vi "lvEtherbone.test_snoop-multi.vi"() -> ()   [LabVIEW 2009, in "lvEtherbone.lvlib"]
doc: "This example performs a multiple read/write _one_ Etherbone device and does this multiple times. This can be used to determine the average time of transactions."
uses:
  lvEtherbone.lvlib
  lvEtherbone.eb_mode_t.ctl
  lvEtherbone.lveb_status_t.ctl
panel:
  out "nOfDevices":i32
  in  "ipPortsFile":path
  out "timePerIteration":dbl=6.0
  in  "nOfIterations":i32=1
  out "timed out?":bool
  out "eb_status":T1
  in  "dataW":u64[](array[numeric])=[291] format="%.0x"
  in  "modeW":T2 items=["EB_UNDEFINED"=-1, "EB_FIFO"=0, "EB_LINEAR"=1]
  in  "addressW":u64=32768 format="%.0x"
  in  "nR":i32
  in  "modeR":T2 items=["EB_UNDEFINED"=-1, "EB_FIFO"=0, "EB_LINEAR"=1]
  out "dataR":u64[](array[numeric]) format="%.0x"
  in  "addressR":u64=32768 format="%.0x"
  in  "timeout [ms]":i32=1000
  out "error out":errorcluster
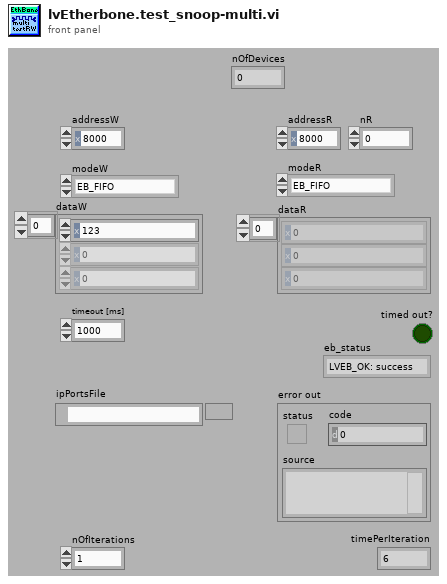
[diagram p1: front panel]
types:
  T1 = typedef "lvEtherbone.lvlib/lvEtherbone.lveb_status_t.ctl" = enum32{"LVEB_OK: success", "LVEB_UNKNOWN: unknown error", "LVEB_OS: operating system forbids access", "LVEB_PORT: port in use or unavailable", "LVEB_ID: ID invalid or out of resources", "LVEB_SOCKET: socket invalid or unavailable", "LVEB_EB: remote address is not Etherbone conformant", "LVEB_IP: bad format or network address", "LVEB_PORTWIDTH: port width error", "LVEB_DEVICEBUSY: Etherbone device still busy", "LVEB_DEVICEFAIL: operation on Wishbone device failed", "LVEB_DEVICEEXIST: Etherbone device already exists, overlaps, or does not exist", "LVEB_TIMEDOUT: a timeout occurred", "LVEB_OVERFLOW: payload of Etherbone exceeded", "LVEB_ADDRESS: bad address", "LVEB_ADDRESSWIDTH: address width error"}
  T2 = typedef "lvEtherbone.lvlib/lvEtherbone.eb_mode_t.ctl" = i32
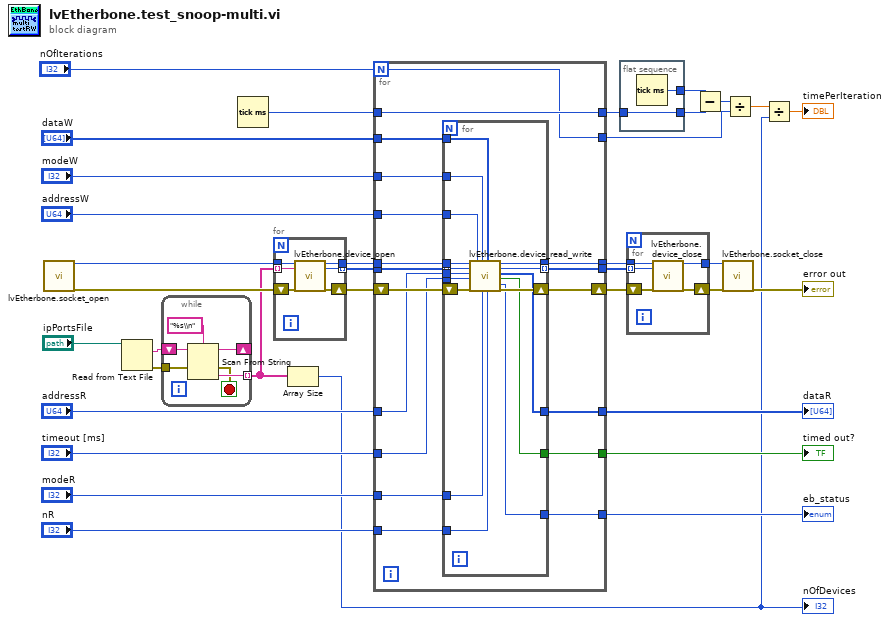
[diagram p0: block diagram]
diagram:
  n1 = call "lvEtherbone.socket_open.vi"() -> ("eb_socket_ID"=w33:i32, "error out"=w34:errorcluster)  [unwired: 17 in, 1 out]
  n2 = Read from Text File(file (use dialog)="ipPortsFile") -> (text=w6:string, error out=w5:errorcluster)  [unwired: 3 in, 2 out]
  n3 = while {
    tunnel: w5 -> [w39]
    tunnel: [w38] -> w2 mode=indexing
    shift-right: [w37] -> _
    shift-left: w6 -> [w41]
    stop <- w36 stop-if-true
    n4 = Scan From String(format string="%s\\n", input string=w41, error in=w39) -> (remaining string=w37:string, error out=w36:errorcluster, output 1=w38:string)  [unwired: 2 in, 1 out]
  }
  n5 = Tick Count (ms)() -> (millisecond timer value=w13:u32)
  n6 = for {
    tunnel: w33 -> [w46]
    tunnel: [w44] -> w30 mode=indexing
    tunnel: [w43] -> w27
    tunnel: w2 -> [w42] mode=indexing
    shift-right: [w45] -> w32
    shift-left: w34 -> [w47]
    n7 = call "lvEtherbone.device_open.vi"("eb_socket_ID"=w46, "ip_port"=w42, "error in (no error)"=w47) -> ("eb_socket_ID out"=w43:i32, "eb_device_ID"=w44:i32, "error out"=w45:errorcluster)  [unwired: 12 in, 2 out]
  }
  n8 = Array Size(array=w2) -> (size(s)=w1:i32)
  "nOfDevices" <- w1
  n9 = for {
    N: "nOfIterations" -> [w48]
    tunnel: w30 -> [w63]
    tunnel: "timeout [ms]" -> [w62]
    tunnel: w27 -> [w61]
    tunnel: [w60] -> w26
    tunnel: [w59] -> w24
    tunnel: "addressR" -> [w58]
    tunnel: [w57] -> w22
    tunnel: "modeR" -> [w56]
    tunnel: "nR" -> [w55]
    tunnel: "addressW" -> [w54]
    tunnel: "modeW" -> [w53]
    tunnel: "dataW" -> [w52]
    tunnel: [w51] -> w16
    tunnel: [w50] -> w15
    tunnel: w13 -> [w49]
    tunnel: [w49] -> w12
    tunnel: [w48] -> w8
    shift-right: [w64] -> w31
    shift-left: w32 -> [w65]
    n10 = for {
      tunnel: w63 -> [w79] mode=indexing
      tunnel: w62 -> [w78]
      tunnel: w61 -> [w77]
      tunnel: [w76] -> w60
      tunnel: [w75] -> w59 mode=indexing
      tunnel: w58 -> [w74]
      tunnel: [w73] -> w57
      tunnel: w56 -> [w72]
      tunnel: w55 -> [w71]
      tunnel: w54 -> [w70]
      tunnel: w53 -> [w69]
      tunnel: w52 -> [w68]
      tunnel: [w67] -> w51
      tunnel: [w66] -> w50
      shift-right: [w80] -> w64
      shift-left: w65 -> [w81]
      n11 = call "lvEtherbone.device_read_write.vi"("eb_socket_ID"=w77, "eb_device_ID"=w79, "addressR"=w74, "timeout [ms]"=w78, "error in (no error)"=w81, "addressW"=w70, "modeW"=w69, "modeR"=w72, "dataW"=w68, "nR"=w71) -> ("eb_status"=w67:T1, "eb_socket_ID out"=w76:i32, "eb_device_ID out"=w75:i32, "dataR"=w73:u64[], "timed out?"=w66:bool, "error out"=w80:errorcluster)  [unwired: 4 in]
    }
  }
  "dataR" <- w22
  "eb_status" <- w16
  "timed out?" <- w15
  n12 = flat-sequence {
    tunnel: w12 -> [w83]
    tunnel: [w83] -> w11
    tunnel: [w82] -> w10
    frame #0 {
      n13 = Tick Count (ms)() -> (millisecond timer value=w82:u32)
    }
  }
  n14 = for {
    tunnel: w26 -> [w86]
    tunnel: [w85] -> w25
    tunnel: w24 -> [w84] mode=indexing
    shift-right: [w87] -> w29
    shift-left: w31 -> [w88]
    n15 = call "lvEtherbone.device_close.vi"("eb_socket_ID"=w86, "eb_device_ID"=w84, "error in (no error)"=w88) -> ("eb_socket_ID out"=w85:i32, "error out"=w87:errorcluster)  [unwired: 14 in, 1 out]
  }
  n16 = Subtract(x=w10, y=w11) -> (x-y=w9:u32)
  n17 = call "lvEtherbone.socket_close.vi"("eb_socket_ID"=w25, "error in (no error)"=w29) -> ("error out"=→"error out":errorcluster)  [unwired: 16 in, 1 out]
  n18 = Divide(x=w9, y=w8) -> (x/y=w3:dbl)
  n19 = Divide(x=w3, y=w1) -> (x/y=→"timePerIteration":dbl)
